vi "8進階題-Three Timer燈.vi"() -> ()   [LabVIEW 2019]
panel:
  in  "Time 3":dbl=10.0 min=0.0 max=10.0 step=0.1 format="%#.1g"
  in  "Time 2":dbl=10.0 min=0.0 max=10.0 step=0.1 format="%#.1g"
  in  "Time 1":dbl=10.0 min=0.0 max=10.0 step=0.1 format="%#.1g"
  out "燈號 3":bool
  in  "按鍵 3":bool
  out "燈號 2":bool
  in  "按鍵 2":bool
  in  "Stop":bool
  out "燈號 1":bool
  in  "按鍵 1":bool
  # "按鍵按下後，燈號依各自設定的時間長度ON之後熄滅\n註：使用一個While Loop，且按鍵按下時，不能有操作Delay的問題"
  # "單位：秒"
  # "單位：秒"
  # "單位：秒"
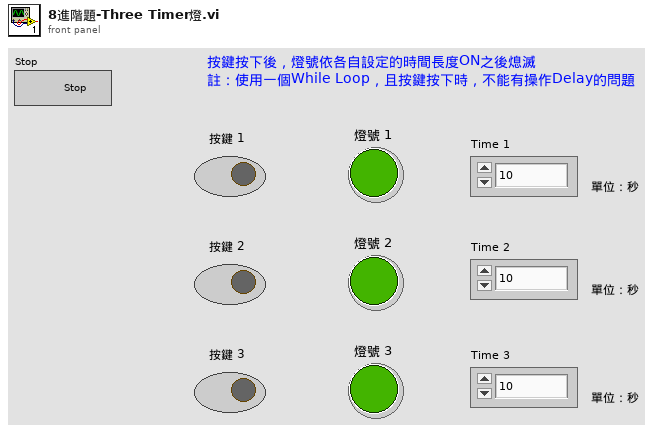
[diagram p1: front panel]
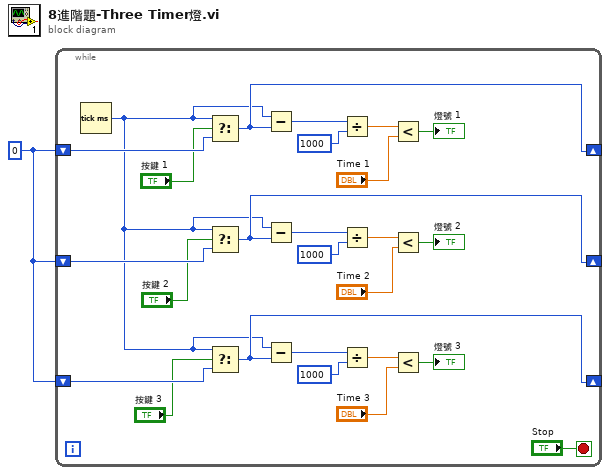
[diagram p0: block diagram]
diagram:
  w1 = u32 0 ("millisecond timer value")
  n1 = while {
    shift-right: [w24] -> _
    shift-left: w1 -> [w27]
    shift-right: [w19] -> _
    shift-left: w1 -> [w18]
    shift-right: [w16] -> _
    shift-left: w1 -> [w17]
    stop <- "Stop" stop-if-true
    n2 = Tick Count (ms)() -> (millisecond timer value=w13:u32)
    n3 = Select(t=w13, s="按鍵 1", f=w27) -> (s? t:f=w24:u32)
    n4 = Select(t=w13, s="按鍵 2", f=w18) -> (s? t:f=w19:u32)
    n5 = Select(t=w13, s="按鍵 3", f=w17) -> (s? t:f=w16:u32)
    n6 = Subtract(x=w13, y=w24) -> (x-y=w23:u32)
    n7 = Subtract(x=w13, y=w19) -> (x-y=w20:u32)
    n8 = Subtract(x=w13, y=w16) -> (x-y=w15:u32)
    n9 = Divide(x=w23, y=u32 1000) -> (x/y=w10:dbl)
    n10 = Divide(x=w20, y=u32 1000) -> (x/y=w7:dbl)
    n11 = Divide(x=w15, y=u32 1000) -> (x/y=w4:dbl)
    n12 = Less?(x=w10, y="Time 1") -> (x < y?=→"燈號 1":bool)
    n13 = Less?(x=w7, y="Time 2") -> (x < y?=→"燈號 2":bool)
    n14 = Less?(x=w4, y="Time 3") -> (x < y?=→"燈號 3":bool)
  }
